vi "2d Gaussian array.vi"(9 "add noise":bool, 10 "multiply A by random number":bool, 11 "A":dbl=4095.0) -> (3 "Intensity Graph":u16[][](graph))   [LabVIEW 2020]
uses:
  NI_PtbyPt.lvlib
panel:
  in  "wx":u8=255
  in  "wy":u8=150
  in  "No spot sizes x":dbl=7.0 format="%.3f"
  out "Numeric 2":i32
  out "Numeric":i32
  in  "only noise":bool
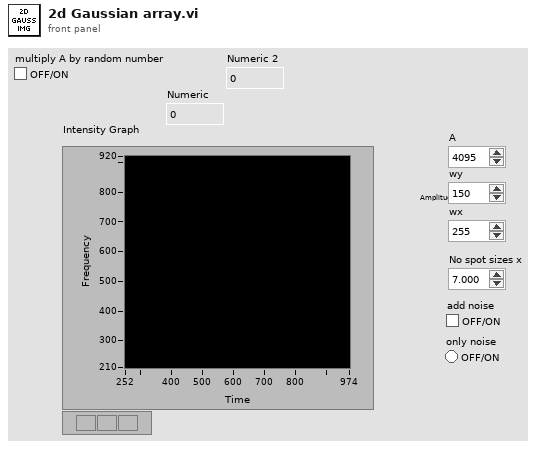
[diagram p1: front panel]
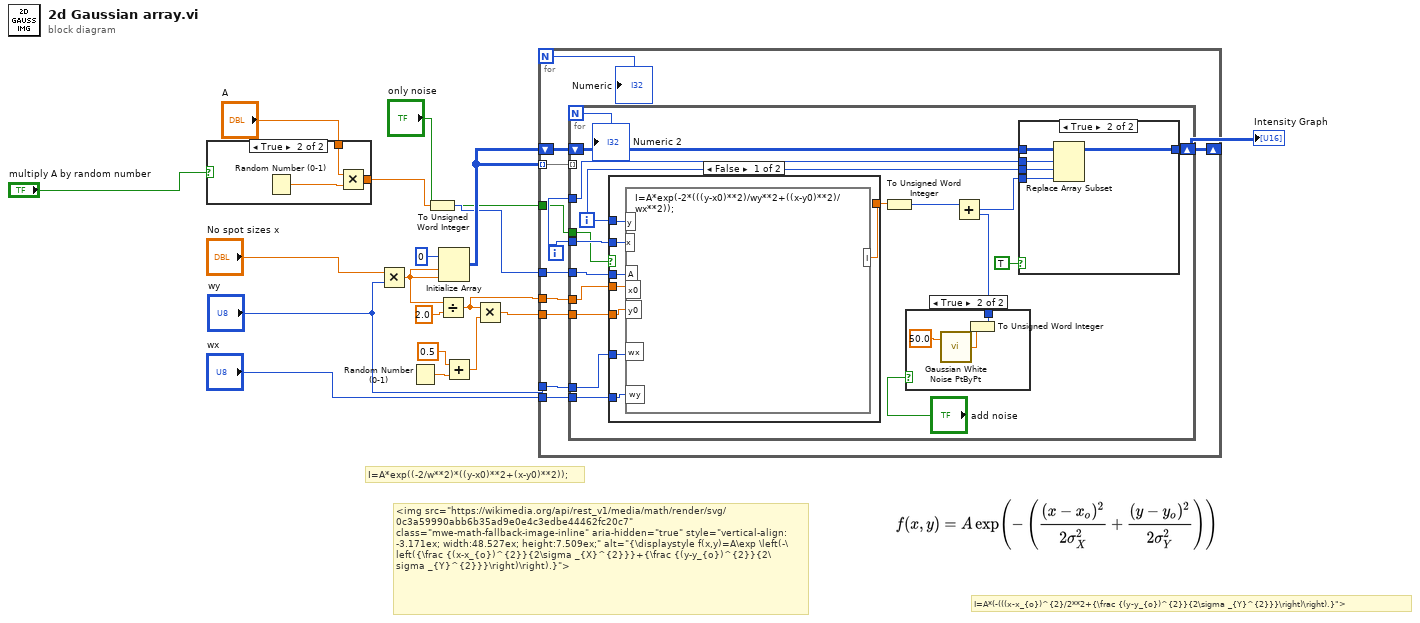
[diagram p0: block diagram]
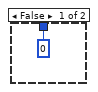
[diagram p3: hidden frame]
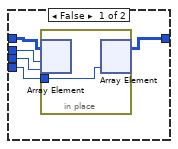
[diagram p4: hidden frame]
diagram:
  # "I=A*(-(((x-x_{o})^{2}/2**2+{\\frac {(y-y_{o})^{2}}{2\\sigma _{Y}^{2}}}\\right)\\right).}\">"
  # "<img src=\"https://wikimedia.org/api/rest_v1/media/math/render/svg/0c3a59990abb6b35ad9e0e4c3edbe44462fc20c7\" class=\"mwe-math-fallback-image-inline\" aria-hidden=\"true\" style=\"vertical-align: -3.171ex; width:48.527ex; height:7.509ex;\" alt=\"{\\displaystyle f(x,y)=A\\exp \\left(-\\left({\\frac {(x-x_{o})^{2}}{2\\sigma _{X}^{2}}}+{\\frac {(y-y_{o})^{2}}{2\\sigma _{Y}^{2}}}\\right)\\right).}\">"
  # "I=A*exp((-2/w**2)*((y-x0)**2+(x-y0)**2));"
  n1 = case shown="True" "multiply A by random number" {
    tunnel: "A" -> [w19 w22]
    tunnel: [w19 w21] -> w5
    frame False {
    }
    frame True {
      n2 = Random Number (0-1)() -> (number: 0 to 1=w20:dbl)
      n3 = Multiply(x=w22, y=w20) -> (x*y=w21:dbl)
    }
  }
  n4 = Multiply(x="No spot sizes x", y="wy") -> (x*y=w8:dbl)
  n5 = Random Number (0-1)() -> (number: 0 to 1=w13:dbl)
  n6 = To Unsigned Word Integer(number=w5) -> (unsigned 16bit integer=w4:u16)
  n7 = Divide(x=w8, y=2.0) -> (x/y=w16:dbl)
  n8 = Initialize Array(u16 0 ("element"), w8, w8) -> (w11:u16[][])
  n9 = Add(x=0.5, y=w13) -> (x+y=w15:dbl)
  n10 = Multiply(x=w16, y=w15) -> (x*y=w17:dbl)
  n11 = for {
    N -> [w24]
    tunnel: w11 -> [w33] mode=indexing
    shift-right: [w31] -> w6
    shift-left: w11 -> [w32]
    tunnel: w4 -> [w30]
    tunnel: w16 -> [w28]
    tunnel: "wy" -> [w27]
    tunnel: w17 -> [w26]
    tunnel: "only noise" -> [w25]
    tunnel: "wx" -> [w23]
    i -> [w29]
    n12 = for {
      N -> [w40]
      tunnel: w33 -> [_] mode=indexing
      shift-right: [w50] -> w31
      shift-left: w32 -> [w51]
      tunnel: w29 -> [w49]
      tunnel: w30 -> [w47]
      tunnel: w29 -> [w46]
      tunnel: w28 -> [w45]
      tunnel: w27 -> [w44]
      tunnel: w26 -> [w43]
      tunnel: w25 -> [w41]
      tunnel: w23 -> [w34]
      i -> [w48]
      n13 = case shown="False" w41 {
        tunnel: w48 -> [w74 _]
        tunnel: w47 -> [w73 _]
        tunnel: w46 -> [w72 _]
        tunnel: w45 -> [w71 _]
        tunnel: w44 -> [w70 _]
        tunnel: w43 -> [w69 _]
        tunnel: [w68 _] -> w37
        tunnel: w34 -> [w67 _]
        frame False {
          n14 = formula code="I=A*exp(-2*(((y-x0)**2)/wy**2+((x-y0)**2)/wx**2));"("y"=w74, "A"=w73, "x0"=w71, "x"=w72, "wx"=w70, "y0"=w69, "wy"=w67) -> ("I"=w68:dbl)
        }
        frame True {
        }
      }
      n15 = To Unsigned Word Integer(number=w37) -> (unsigned 16bit integer=w36:u16)
      n16 = case shown="True" "add noise" {
        tunnel: [u16 0 w53] -> w38
        frame False {
        }
        frame True {
          n17 = call "Gaussian White Noise PtByPt.vi"("standard deviation"=50.0) -> ("Gaussian white noise"=w54:dbl)  [unwired: 2 in]
          n18 = To Unsigned Word Integer(number=w54) -> (unsigned 16bit integer=w53:u16)
        }
      }
      n19 = Add(x=w36, y=w38) -> (x+y=w42:u16)
      n20 = case shown="True" TRUE {
        tunnel: w51 -> [w60 w66]
        tunnel: [w59 w65] -> w50
        tunnel: w49 -> [w58 w64]
        tunnel: w48 -> [w57 w63]
        tunnel: w42 -> [w56 w62]
        frame False {
          n21 = in-place {
            in-place-border: w56 -> [w61]
            n22 = in-place-array #1(w60, w58, w57) -> ()  [unwired: 1 out]
            n23 = in-place-array #1(w61) -> (w59:u16[][])  [unwired: 2 out]
          }
        }
        frame True {
          n24 = Replace Array Subset(array=w66, new element=w62, index (row)=w64, index (col)=w63) -> (w65:u16[][])
        }
      }
      "Numeric 2" <- w40
    }
    "Numeric" <- w24
  }
  "Intensity Graph" <- w6
